vi "From String.vi"(8 "error in (no error)":errorcluster, 9 "initial scan location":u32, 10 "String":string, 11 "Type in":refnum<class "Abs_Boolean_1D.lvclass">) -> (0 "error out":errorcluster, 1 "offset past scan":u32, 2 "Remaining String":string, 3 "Type out":refnum<class "Abs_Boolean_1D.lvclass">)   [LabVIEW 2021, in "Abs_Boolean_1D.lvclass"]
uses:
  Abs_Boolean_1D.lvclass
  Abs_Boolean_1D.lvclass/Abs_Boolean_1D.ctl
  Properties/Read From String Match.vi
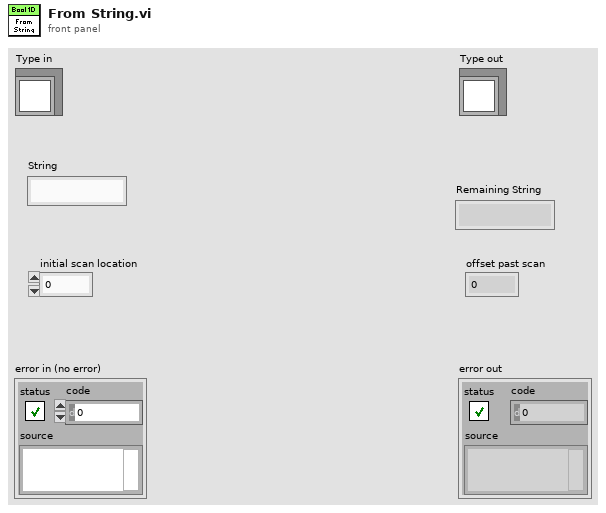
[diagram p1: front panel]
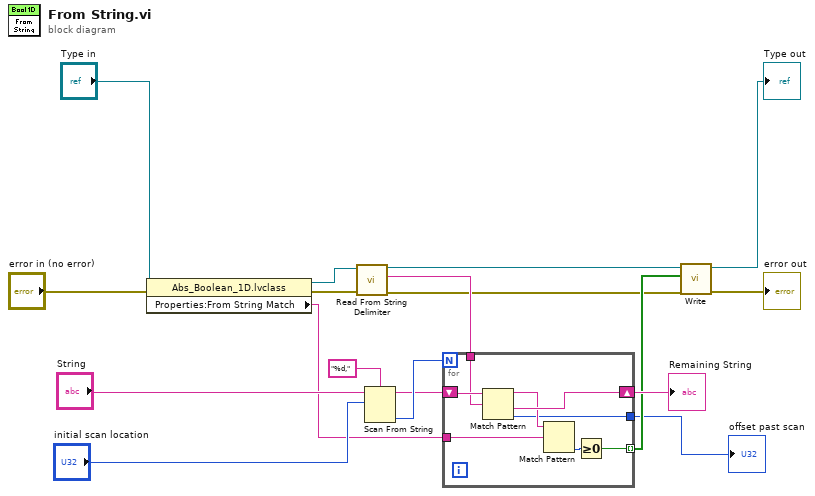
[diagram p0: block diagram]
diagram:
  n1 = property class="Abs_Boolean_1D.lvclass"(reference="Type in", error in="error in (no error)") -> (reference out=w4:refnum<class "Abs_Boolean_1D.lvclass">, error out=w5:errorcluster, "Properties:From String Match"=w8:string)
  n2 = call-dynamic "Read From String Delimiter.vi"("error in (no error)"=w5, "Abs_Array in"=w4) -> ("error out"=w2:errorcluster, "From String Delimiter"=w3:string, "Abs_Array out"=w1:refnum<class "Abs_Boolean_1D.lvclass">)  [unwired: 7 in]
  n3 = Scan From String(format string="%d,", input string="String", initial scan location="initial scan location") -> (remaining string=w11:string, output 1=w12:i32)  [unwired: 2 in, 2 out]
  n4 = for {
    N: w12 -> [_]
    shift-right: [w24] -> w10
    shift-left: w11 -> [w26]
    tunnel: w3 -> [w25]
    tunnel: w8 -> [w21]
    tunnel: [w20] -> w7 mode=indexing
    tunnel: [w19] -> w6
    n5 = Match Pattern(string=w26, regular expression=w25) -> (before substring=w22:string, after substring=w24:string, offset past match=w19:i32)  [unwired: 1 in, 1 out]
    n6 = Match Pattern(string=w22, regular expression=w21) -> (offset past match=w23:i32)  [unwired: 1 in, 3 out]
    n7 = Greater Or Equal To 0?(x=w23) -> (x >= 0?=w20:bool)
  }
  "Remaining String" <- w10
  "offset past scan" <- w6
  n8 = call-dynamic "Write.vi"("error in (no error)"=w2, "Boolean 1D"=w7, "Boolean in"=w1) -> ("error out"=→"error out":errorcluster, "Boolean out"=→"Type out":refnum<class "Abs_Boolean_1D.lvclass">)  [unwired: 7 in]
